vi "Update.vi"(8 "error in (no error)":errorcluster, 9 "EQ VI Ref":refnum<vi>, 10 "Audio Block In":dbl[][](array[numeric]), 11 "Channel in":refnum<class "Channel.lvclass">) -> (0 "error out":errorcluster, 1 "Headphones Audio Block Out":dbl[][](array[numeric]), 2 "Master Audio Block Out":dbl[][](array[numeric]), 3 "Channel out":refnum<class "Channel.lvclass">)   [LabVIEW 2020, in "Channel.lvclass"]
uses:
  Channel.lvclass
  Channel.lvclass/Channel.ctl
  Packed Libraries/Globals.lvlibp/Constants.vi
  Packed Libraries/Globals.lvlibp
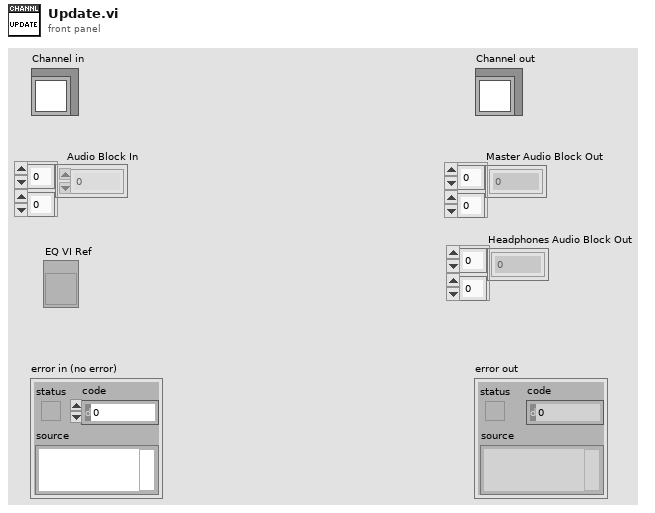
[diagram p1: front panel]
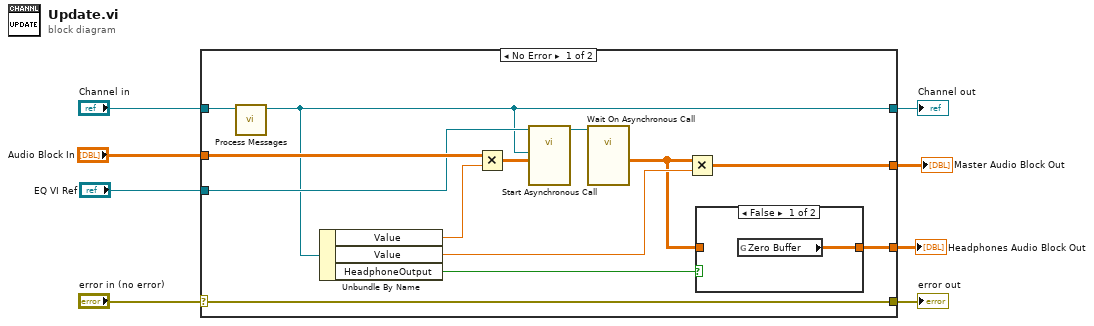
[diagram p0: block diagram]
diagram:
  n1 = case shown="No Error" "error in (no error)" {
    selector: "error in (no error)" -> [w21 w26]
    tunnel: [w21 w26] -> w7
    tunnel: [w9 w25] -> w5
    tunnel: "Channel in" -> [w13 w25]
    tunnel: [w18 w24] -> w4
    tunnel: "Audio Block In" -> [w14 w24]
    tunnel: [w16 w24] -> w2
    tunnel: "EQ VI Ref" -> [w12 _]
    frame No Error {
      n2 = call "Process Messages.vi"("Channel in"=w13) -> ("Channel out"=w9:refnum<class "Channel.lvclass">)  [unwired: 9 in, 1 out]
      n3 = Unbundle By Name(w9) -> ("Value"=w20:dbl, "Value"=w19:dbl, "HeadphoneOutput"=w17:bool)
      n4 = Multiply(x=w14, y=w20) -> (x*y=w10:dbl[][])
      n5 = call-by-ref "Start Asynchronous Call"(reference=w12, "Audio Block In"=w10, "Channel in"=w9) -> (reference out=w11:refnum<vi>)  [unwired: 9 in, 3 out]
      n6 = call-by-ref "Wait On Asynchronous Call"(reference=w11) -> ("Audio Block Out"=w15:dbl[][])  [unwired: 11 in, 3 out]
      n7 = Multiply(x=w15, y=w19) -> (x*y=w18:dbl[][])
      n8 = case shown="False" w17 {
        tunnel: [w22 w23] -> w16
        tunnel: w15 -> [_ w23]
        frame False {
          n9 = global read "Constants.vi" "Zero Buffer"() -> (w22:dbl[][])
        }
        frame True {
        }
      }
    }
    frame Error {
    }
  }
  "error out" <- w7
  "Channel out" <- w5
  "Master Audio Block Out" <- w4
  "Headphones Audio Block Out" <- w2
